vi "Get New Mentions - Continuous.vi"() -> ()   [LabVIEW 2011]
doc: "This example gets new mentions that were posted since the last call to this VI continuously. If mentions are posted after a call to Get New Mentions.vi, the next call to Get New Mentions.vi will get the newest mentions since the last call to Get New Mentions.vi."
uses:
  Controls/Tweet.ctl
  i3-twitter.lvlib
panel:
  out "Mentions Read":T1[](array[typedef])
  in  "stop":bool
  out "Time Stamp of Newest Mentions":timestamp
  out "Num of Mentions Read":i32
  in  "Num of Mentions to Read":i32
  in  "Consumer Key":string
  in  "Consumer Secret":string
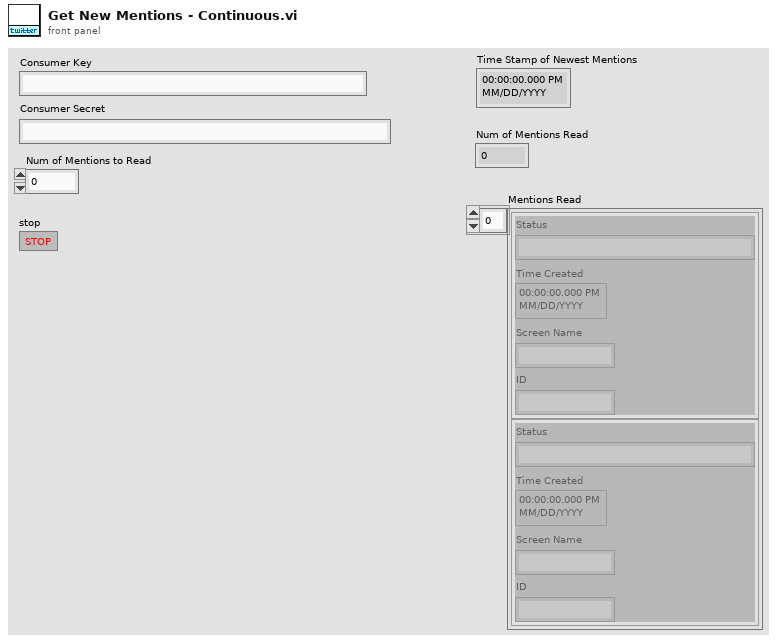
[diagram p1: front panel]
types:
  T1 = typedef "i3-twitter.lvlib/Tweet.ctl" = cluster{"Status":string, "Time Created":timestamp, "Screen Name":string, "ID":string}
  T2 = typedef "i3-twitter.lvlib/Twitter Handle.ctl" = cluster{"OAuth Credentials":T3, "since ID":string, "max ID":string, "Screen Name":string}
  T3 = typedef "i3-oauth.lvlib/OAuth Credentials.ctl" = cluster{"Consumer Key":string, "Signature Method":T4, "Token":string, "Version":string, "Token Secret":string, "Consumer Secret":string}
  T4 = typedef "i3-oauth.lvlib/Signature Method.ctl" = enum16{"HMAC-MD5", "HMAC-SHA1", "HMAC-SHA224", "HMAC-SHA256", "HMAC-SHA384", "HMAC-SHA512"}
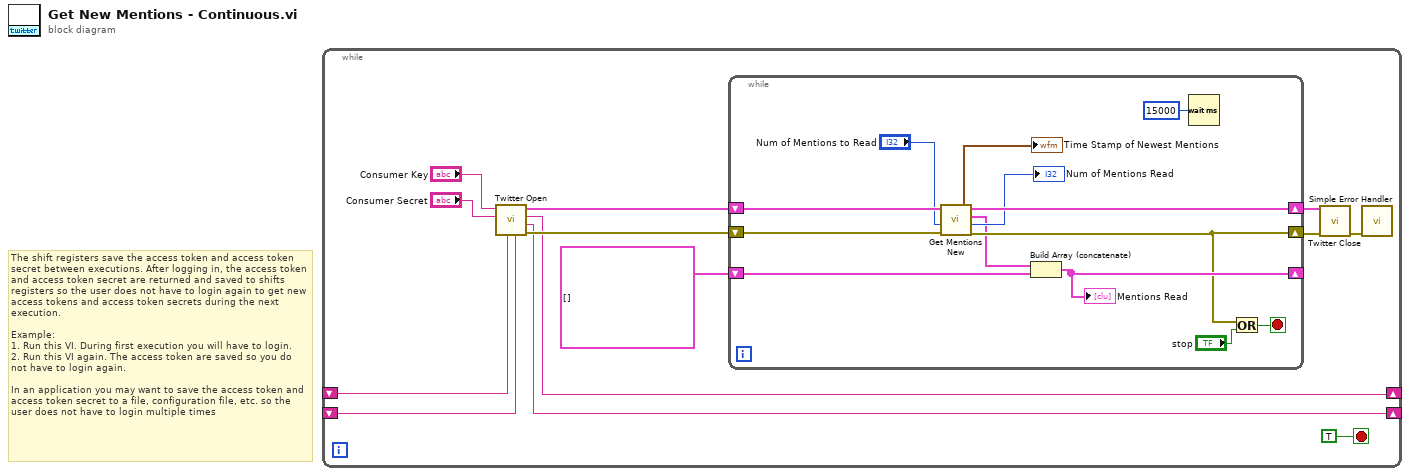
[diagram p0: block diagram]
diagram:
  # "The shift registers save the access token and access token secret between executions. After logging in, the access token and access token secret are returned and saved to shifts registers so the user does not have to login again to get new access tokens and access token secrets during the next execution.\n\nExample:\n1. Run this VI. During first execution you will have to login.\n2. Run this VI again. The access token are saved so you do not have to login again.\n\nIn an application you may want to save the access token and access token secret to a file, configuration file, etc. so the user does not have to login multiple times"
  n1 = while {
    shift-right: [w4] -> _
    shift-left: _ -> [w2]
    shift-right: [w3] -> _
    shift-left: _ -> [w1]
    stop <- TRUE stop-if-true
    n2 = call "Twitter Open.vi"("Access Token Secret (In)"=w1, "Access Token (In)"=w2, "Consumer Secret"="Consumer Secret", "Consumer Key"="Consumer Key") -> ("error out"=w7:errorcluster, "Access Token Secret (Out)"=w3:string, "Access Token (Out)"=w4:string, "Twitter Handle Out"=w11:T2)  [unwired: 4 in]
    n3 = while {
      shift-right: [w24] -> w9
      shift-left: w11 -> [w26]
      shift-right: [w22] -> _
      shift-left: T1[] [] ("Tweets Array") -> [w15]
      shift-right: [w19] -> w10
      shift-left: w7 -> [w25]
      stop <- w18 stop-if-true
      n4 = call "Get Mentions New.vi"("error in"=w25, "Mentions to Read (10)"="Num of Mentions to Read", "Twitter Handle In"=w26) -> ("error out"=w19:errorcluster, "Actual Num of Mentions Read"=→"Num of Mentions Read":i32, "New Mentions Read"=w16:T1[], "Twitter Handle Out"=w24:T2, "Time Stamp of Newest Mention"=→"Time Stamp of Newest Mentions":timestamp)  [unwired: 4 in]
      n5 = Build Array (concatenate)(w16, w15) -> (w22:T1[])
      "Mentions Read" <- w22
      n6 = Wait (ms)(milliseconds to wait=u32 15000) -> ()  [unwired: 1 out]
      n7 = Or(x=w19, y="stop") -> (x .or. y?=w18:bool)
    }
    n8 = call "Twitter Close.vi"("error in"=w10, "Twitter Handle In"=w9) -> ("error in"=w5:errorcluster)  [unwired: 9 in]
    n9 = call <vilib>:"Simple Error Handler.vi"("error in (no error)"=w5) -> ()  [unwired: 4 in, 5 out]
  }
